vi "Read_raw_meas_setup.vi"(8 "Setup file string":string) -> (0 "No of Blocks":i32=1, 1 "Sampling freq (Hz)":dbl=100.0, 2 "No of samples":i32=500 min=0 step=1, 3 "Position":T2(array[cluster])=[{"Name"="LDA  (U)", "X"=3650.0, "Y"=0.0, "Z"=47.5}, {"Name"="Pitot 1 (Upitot)", "X"=3110.0, "Y"=0.0, "Z"=450.0}] {"Z" format="%.1f"; "Y" format="%.1f"; "X" format="%.1f"}, 5 "Correlate?":T1(ring))   [LabVIEW 2010]
uses:
  Globals/Meas_global.vi
  Globals/Trav_pos_global.vi
  Globals/LDA_meas_global_1.vi
  Globals/LDA_meas_global_2.vi
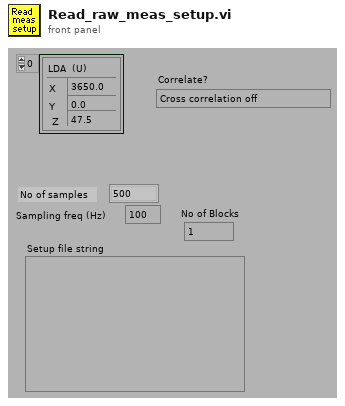
[diagram p1: front panel]
types:
  T1 = enum16{"Cross correlation off", "Show correlation panel", "Correlate without activating panel"}
  T2 = cluster{"Name":string, "X":dbl, "Y":dbl, "Z":dbl}[]
  T3 = typedef "Post_Process.ctl" = enum16{"Take New Data", "Post Process Raw Data File"}
  T4 = cluster{"Name":string, "X":dbl, "Y":dbl, "Z":dbl}
  T5 = enum16{"To Traverse Coordinates", "To User Coordinates"}
  T6 = enum16{"From String to Cluster", "From Cluster to String"}
  T7 = typedef "BSA_Type.ctl" = enum16{"57N11", "BSA F60"}
  T8 = typedef "BSA_info_Cluster.ctl" = cluster{"GPIB Address":string, "No of Check Bytes":i32, "Extra Info":string, "COLOUR":u32, "Wavelength (nm)":dbl}
  T9 = typedef "Tunnel_Coordinates.ctl" = enum16{"Work in Tunnel Coordinates", "Work in Model Coordinates"}
  T10 = typedef "Graph_Type.ctl" = enum16{"Show no graph", "Voltage trace", "Velocity trace", "Vel histogram", "Spectrum", "f.E(f) v Log f", "Auto-Corr"}
  T11 = cluster{"Plot 1":u16, "Plot 2":u16, "Save graph":u16, "Plot Type":T10}
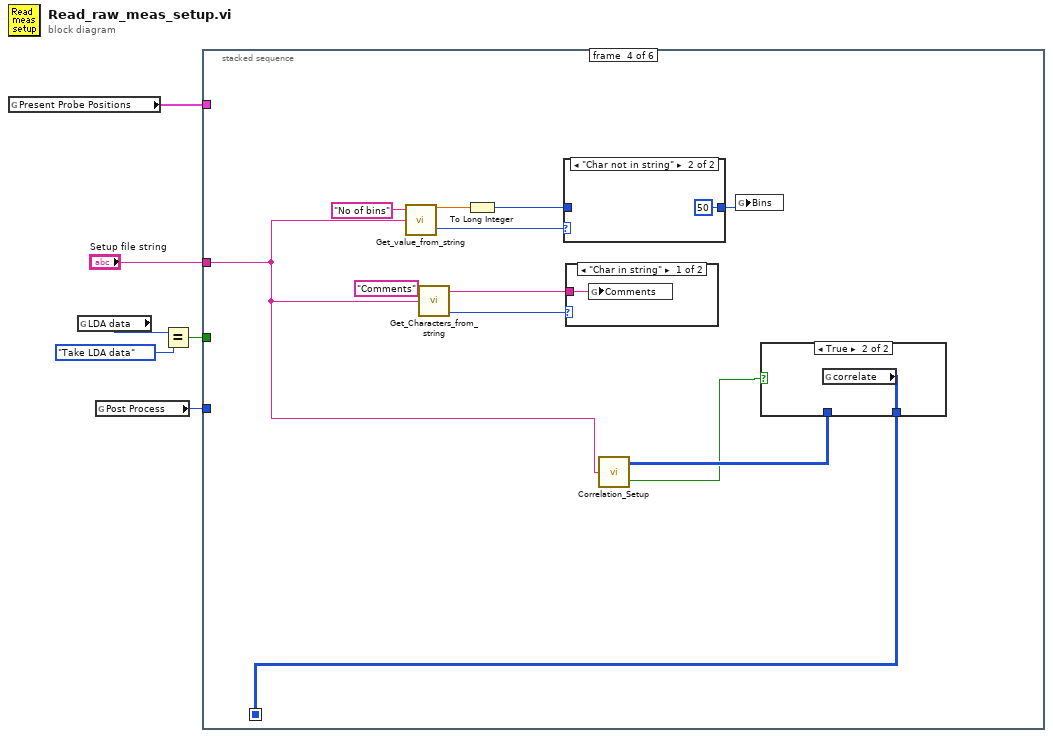
[diagram p0: block diagram]
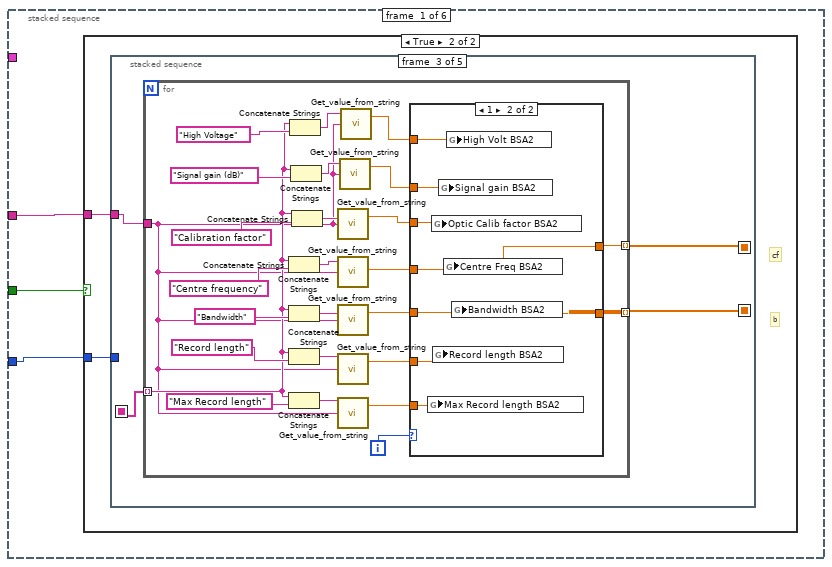
[diagram p2: hidden frame]
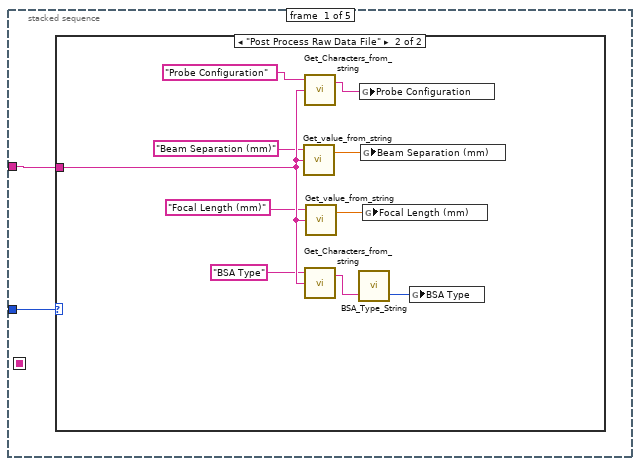
[diagram p4: hidden frame]
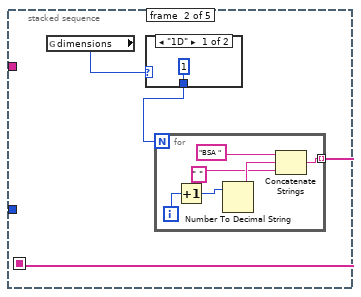
[diagram p6: hidden frame]
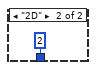
[diagram p7: hidden frame]
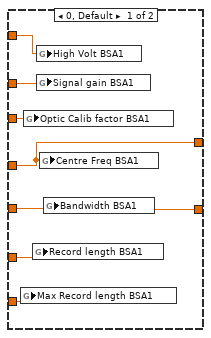
[diagram p8: hidden frame]
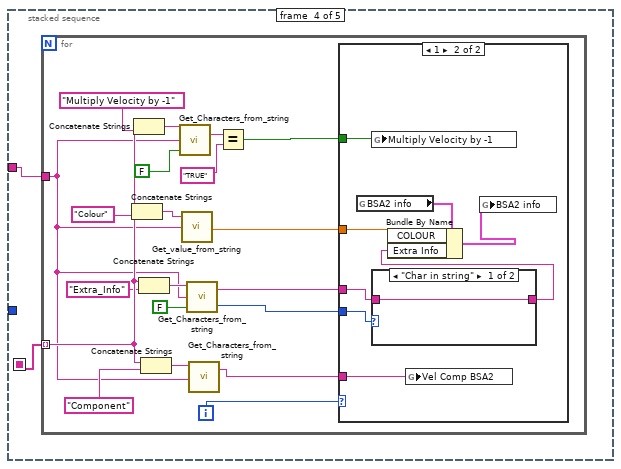
[diagram p9: hidden frame]
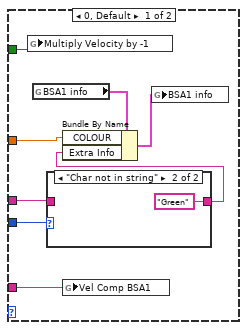
[diagram p10: hidden frame]
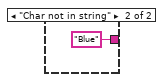
[diagram p12: hidden frame]
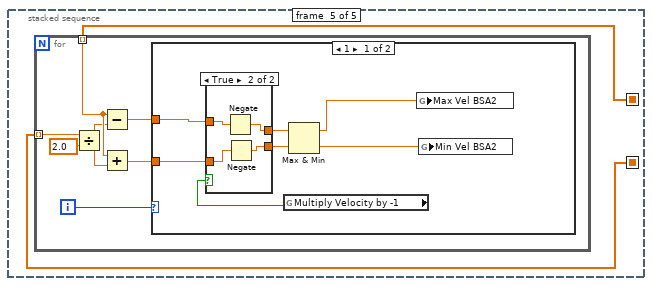
[diagram p13: hidden frame]
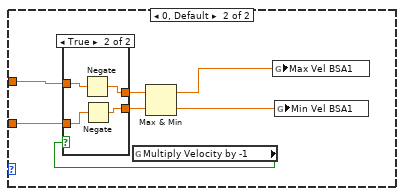
[diagram p15: hidden frame]
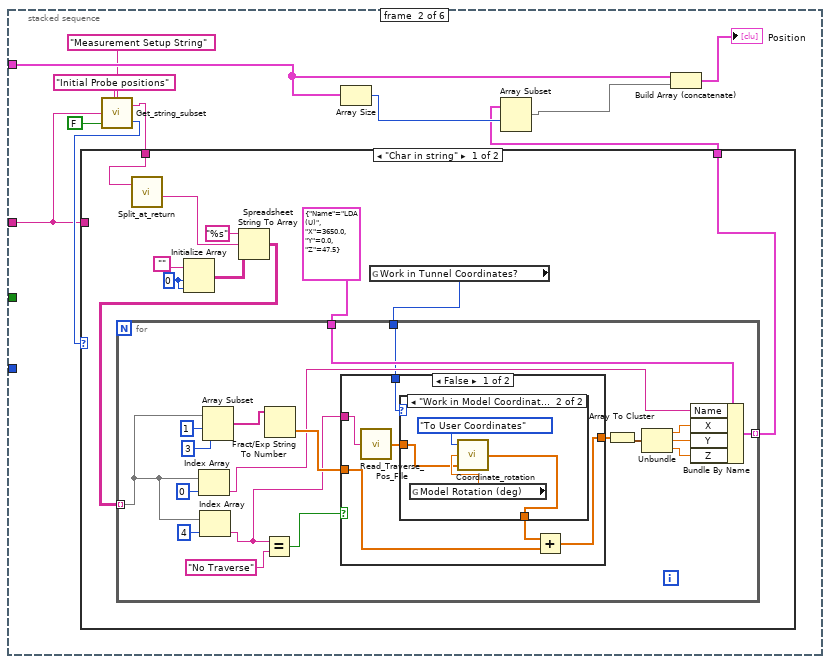
[diagram p17: hidden frame]
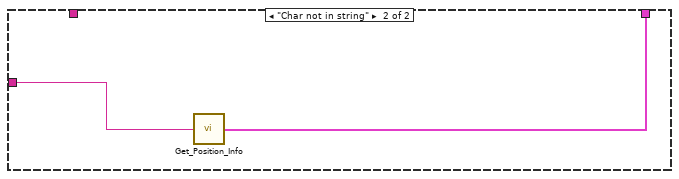
[diagram p20: hidden frame]
diagram:
  n1 = global read "Trav_pos_global.vi" "Present Probe Positions"() -> (w5:T2)
  n2 = global read "Meas_global.vi" "LDA data"() -> (w3:enum16{"No LDA data", "Take LDA data"})
  n3 = global read "Meas_global.vi" "Post Process"() -> (w6:T3)
  n4 = Equal?(x=w3, y=enum16{"No LDA data", "Take LDA data"}."Take LDA data" ("LDA data")) -> (x = y?=w2:bool)
  n5 = stacked-sequence {
    seq-local: [_ _ _ w226 _ _] -> [_ _ _ _ w245 _]
    tunnel: w6 -> [w7 _ _ _ _ _]
    tunnel: w5 -> [_ w165 _ _ _ _]
    tunnel: w2 -> [w9 _ _ _ _ _]
    tunnel: "Setup file string" -> [w8 w157 w215 w223 _ w248]
    frame #0 {
      n6 = case shown="True" w9 {
        tunnel: w8 -> [_ w11]
        tunnel: w7 -> [_ w10]
        frame False {
        }
        frame True {
          # "b"
          # "cf"
          n7 = stacked-sequence {
            seq-local: [_ w24 _ _ _] -> [_ _ w37 w79 _]
            seq-local: [_ _ w35 _ _] -> [_ _ _ _ w121]
            seq-local: [_ _ w36 _ _] -> [_ _ _ _ w122]
            tunnel: w11 -> [w12 _ w38 w80 _]
            tunnel: w10 -> [w13 _ _ _ _]
            frame #0 {
              n8 = case shown="\"Post Process Raw Data File\"" w13 {
                tunnel: w12 -> [_ w21]
                frame "Take New Data" {
                }
                frame "Post Process Raw Data File" {
                  n9 = call "Get_value_from_string.vi"("Input string"=w21, "Variable name"="Beam Separation (mm)" ("Label for characters")) -> ("Value"=w14:dbl)  [unwired: 1 in, 1 out]
                  n10 = call "Get_Characters_from_string.vi"("Input string"=w21, "Variable name"="Probe Configuration" ("Label for characters")) -> ("Value"=w22:string)  [unwired: 1 in, 1 out]
                  n11 = call "Get_Characters_from_string.vi"("Input string"=w21, "Variable name"="BSA Type" ("Label for characters")) -> ("Value"=w17:string)  [unwired: 1 in, 1 out]
                  n12 = call "Get_value_from_string.vi"("Input string"=w21, "Variable name"="Focal Length (mm)" ("Label for characters")) -> ("Value"=w15:dbl)  [unwired: 1 in, 1 out]
                  n13 = call "BSA_Type_String.vi"("BSA String in"=w17) -> ("BSA Type Out"=w16:T7)  [unwired: 1 in, 1 out]
                  n14 = global write "LDA_meas_global_1.vi" "Probe Configuration"(w22) -> ()
                  n15 = global write "LDA_meas_global_1.vi" "Beam Separation (mm)"(w14) -> ()
                  n16 = global write "LDA_meas_global_1.vi" "Focal Length (mm)"(w15) -> ()
                  n17 = global write "LDA_meas_global_1.vi" "BSA Type"(w16) -> ()
                }
              }
            }
            frame #1 {
              n18 = global read "Meas_global.vi" "dimensions"() -> (w26:enum16{"1D", "2D"})
              n19 = case shown="\"1D\"" w26 {
                tunnel: [1 2] -> w25
                frame "1D" {
                }
                frame "2D" {
                }
              }
              n20 = for {
                N: w25 -> [_]
                tunnel: [w28] -> w24 mode=indexing
                i -> [w30]
                n21 = Increment(x=w30) -> (x+1=w29:i32)
                n22 = Number To Decimal String(number=w29) -> (decimal integer string=w32:string)  [unwired: 1 out]
                n23 = Concatenate Strings("BSA ", w32, " ") -> (w28:string)
              }
            }
            frame #2 {
              n24 = for {
                tunnel: w38 -> [w39]
                tunnel: w37 -> [w40] mode=indexing
                tunnel: [w52] -> w36 mode=indexing
                tunnel: [w51] -> w35 mode=indexing
                i -> [w56]
                n25 = Concatenate Strings(w40, "Centre frequency") -> (w59:string)
                n26 = Concatenate Strings(w40, "Bandwidth") -> (w58:string)
                n27 = Concatenate Strings(w40, "Record length") -> (w57:string)
                n28 = Concatenate Strings(w40, "Max Record length") -> (w42:string)
                n29 = Concatenate Strings(w40, "High Voltage") -> (w46:string)
                n30 = Concatenate Strings(w40, "Signal gain (dB)") -> (w47:string)
                n31 = Concatenate Strings(w40, "Calibration factor") -> (w60:string)
                n32 = call "Get_value_from_string.vi"("Input string"=w39, "Variable name"=w60) -> ("Value"=w50:dbl)  [unwired: 1 in, 1 out]
                n33 = call "Get_value_from_string.vi"("Input string"=w39, "Variable name"=w59) -> ("Value"=w55:dbl)  [unwired: 1 in, 1 out]
                n34 = call "Get_value_from_string.vi"("Input string"=w39, "Variable name"=w58) -> ("Value"=w54:dbl)  [unwired: 1 in, 1 out]
                n35 = call "Get_value_from_string.vi"("Input string"=w39, "Variable name"=w57) -> ("Value"=w53:dbl)  [unwired: 1 in, 1 out]
                n36 = call "Get_value_from_string.vi"("Input string"=w39, "Variable name"=w42) -> ("Value"=w43:dbl)  [unwired: 1 in, 1 out]
                n37 = call "Get_value_from_string.vi"("Input string"=w39, "Variable name"=w47) -> ("Value"=w45:dbl)  [unwired: 1 in, 1 out]
                n38 = call "Get_value_from_string.vi"("Input string"=w39, "Variable name"=w46) -> ("Value"=w44:dbl)  [unwired: 1 in, 1 out]
                n39 = case shown="1" w56 {
                  tunnel: w55 -> [w68 w76]
                  tunnel: w54 -> [w69 w75]
                  tunnel: w53 -> [w70 w78]
                  tunnel: w50 -> [w71 w77]
                  tunnel: [w69 w75] -> w52
                  tunnel: [w68 w76] -> w51
                  tunnel: w45 -> [w67 w73]
                  tunnel: w44 -> [w66 w74]
                  tunnel: w43 -> [w65 w72]
                  frame 0, Default {
                    n40 = global write "LDA_meas_global_1.vi" "Max Record length BSA1"(w65) -> ()
                    n41 = global write "LDA_meas_global_1.vi" "Optic Calib factor BSA1"(w71) -> ()
                    n42 = global write "LDA_meas_global_1.vi" "Record length BSA1"(w70) -> ()
                    n43 = global write "LDA_meas_global_1.vi" "High Volt BSA1"(w66) -> ()
                    n44 = global write "LDA_meas_global_1.vi" "Signal gain BSA1"(w67) -> ()
                    n45 = global write "LDA_meas_global_1.vi" "Centre Freq BSA1"(w68) -> ()
                    n46 = global write "LDA_meas_global_1.vi" "Bandwidth BSA1"(w69) -> ()
                  }
                  frame 1 {
                    n47 = global write "LDA_meas_global_2.vi" "Max Record length BSA2"(w72) -> ()
                    n48 = global write "LDA_meas_global_2.vi" "Optic Calib factor BSA2"(w77) -> ()
                    n49 = global write "LDA_meas_global_2.vi" "Record length BSA2"(w78) -> ()
                    n50 = global write "LDA_meas_global_2.vi" "Signal gain BSA2"(w73) -> ()
                    n51 = global write "LDA_meas_global_2.vi" "Centre Freq BSA2"(w76) -> ()
                    n52 = global write "LDA_meas_global_2.vi" "High Volt BSA2"(w74) -> ()
                    n53 = global write "LDA_meas_global_2.vi" "Bandwidth BSA2"(w75) -> ()
                  }
                }
              }
            }
            frame #3 {
              n54 = for {
                tunnel: w80 -> [w81]
                tunnel: w79 -> [w86] mode=indexing
                i -> [w98]
                n55 = Concatenate Strings(w86, "Colour") -> (w99:string)
                n56 = Concatenate Strings(w86, "Multiply Velocity by -1") -> (w92:string)
                n57 = Concatenate Strings(w86, "Extra_Info" ("string")) -> (w87:string)
                n58 = Concatenate Strings(w86, "Component") -> (w100:string)
                n59 = call "Get_Characters_from_string.vi"("Show Dialog?"=FALSE, "Input string"=w81, "Variable name"=w92) -> ("Value"=w90:string)  [unwired: 1 out]
                n60 = call "Get_value_from_string.vi"("Input string"=w81, "Variable name"=w99) -> ("Value"=w95:dbl)  [unwired: 1 in, 1 out]
                n61 = call "Get_Characters_from_string.vi"("Show Dialog?"=FALSE, "Input string"=w81, "Variable name"=w87) -> ("Status"=w83:enum16{"Char in string", "Char not in string"}, "Value"=w82:string)
                n62 = call "Get_Characters_from_string.vi"("Input string"=w81, "Variable name"=w100) -> ("Value"=w94:string)  [unwired: 1 in, 1 out]
                n63 = Equal?(x=w90, y="TRUE") -> (x = y?=w88:bool)
                n64 = case shown="1" w98 {
                  tunnel: w95 -> [w107 w117]
                  tunnel: w94 -> [w106 w116]
                  tunnel: w88 -> [w105 w115]
                  tunnel: w83 -> [w104 w112]
                  tunnel: w82 -> [w103 w113]
                  frame 0, Default {
                    n65 = global write "LDA_meas_global_1.vi" "Multiply Velocity by -1"(w105) -> ()
                    n66 = global read "LDA_meas_global_1.vi" "BSA1 info"() -> (w108:T8)
                    n67 = case shown="\"Char not in string\"" w104 {
                      tunnel: w103 -> [w109 _]
                      tunnel: [w109 "Green" ("Value")] -> w101
                      frame "Char in string" {
                      }
                      frame "Char not in string" {
                      }
                    }
                    n68 = Bundle By Name(cluster=w108, "COLOUR"=w107, "Extra Info"=w101) -> (w102:T8)
                    n69 = global write "LDA_meas_global_1.vi" "Vel Comp BSA1"(w106) -> ()
                    n70 = global write "LDA_meas_global_1.vi" "BSA1 info"(w102) -> ()
                  }
                  frame 1 {
                    n71 = global read "LDA_meas_global_2.vi" "BSA2 info"() -> (w118:T8)
                    n72 = global write "LDA_meas_global_2.vi" "Multiply Velocity by -1"(w115) -> ()
                    n73 = case shown="\"Char in string\"" w112 {
                      tunnel: w113 -> [w119 _]
                      tunnel: [w119 "Blue" ("Value")] -> w111
                      frame "Char in string" {
                      }
                      frame "Char not in string" {
                      }
                    }
                    n74 = Bundle By Name(cluster=w118, "COLOUR"=w117, "Extra Info"=w111) -> (w114:T8)
                    n75 = global write "LDA_meas_global_2.vi" "Vel Comp BSA2"(w116) -> ()
                    n76 = global write "LDA_meas_global_2.vi" "BSA2 info"(w114) -> ()
                  }
                }
              }
            }
            frame #4 {
              n77 = for {
                tunnel: w122 -> [w128] mode=indexing
                tunnel: w121 -> [w127] mode=indexing
                i -> [w123]
                n78 = Divide(x=w128, y=2.0) -> (x/y=w126:dbl)
                n79 = Subtract(x=w127, y=w126) -> (x-y=w124:dbl)
                n80 = Add(x=w127, y=w126) -> (x+y=w125:dbl)
                n81 = case shown="1" w123 {
                  tunnel: w125 -> [w136 w149]
                  tunnel: w124 -> [w135 w148]
                  frame 1 {
                    n82 = global read "LDA_meas_global_2.vi" "Multiply Velocity by -1"() -> (w132:bool)
                    n83 = case shown="True" w132 {
                      tunnel: w136 -> [w137 w142]
                      tunnel: w135 -> [w138 w141]
                      tunnel: [w138 w140] -> w134
                      tunnel: [w137 w139] -> w133
                      frame False {
                      }
                      frame True {
                        n84 = Negate(x=w141) -> (-x=w140:dbl)
                        n85 = Negate(x=w142) -> (-x=w139:dbl)
                      }
                    }
                    n86 = Max & Min(x=w134, y=w133) -> (max(x,y)=w130:dbl, min(x,y)=w131:dbl)
                    n87 = global write "LDA_meas_global_2.vi" "Max Vel BSA2"(w130) -> ()
                    n88 = global write "LDA_meas_global_2.vi" "Min Vel BSA2"(w131) -> ()
                  }
                  frame 0, Default {
                    n89 = global read "LDA_meas_global_1.vi" "Multiply Velocity by -1"() -> (w145:bool)
                    n90 = case shown="True" w145 {
                      tunnel: w149 -> [w150 w155]
                      tunnel: w148 -> [w151 w154]
                      tunnel: [w151 w153] -> w147
                      tunnel: [w150 w152] -> w146
                      frame False {
                      }
                      frame True {
                        n91 = Negate(x=w154) -> (-x=w153:dbl)
                        n92 = Negate(x=w155) -> (-x=w152:dbl)
                      }
                    }
                    n93 = Max & Min(x=w147, y=w146) -> (max(x,y)=w143:dbl, min(x,y)=w144:dbl)
                    n94 = global write "LDA_meas_global_1.vi" "Max Vel BSA1"(w143) -> ()
                    n95 = global write "LDA_meas_global_1.vi" "Min Vel BSA1"(w144) -> ()
                  }
                }
              }
            }
          }
        }
      }
    }
    frame #1 {
      n96 = call "Get_string_subset.vi"("String Name"="Measurement Setup String", "Show Dialog?"=FALSE, "String to split"=w157, "File Label"="Initial Probe positions") -> ("Status"=w162:enum16{"Char in string", "Char not in string"}, "Output string"=w161:string)
      n97 = case shown="\"Char in string\"" w162 {
        tunnel: w161 -> [w172 _]
        tunnel: w157 -> [_ w209]
        tunnel: [w168 w208] -> w159
        frame "Char in string" {
          w175 = 0 ("Dimension Size")
          n98 = call "Split_at_return.vi"("String"=w172) -> ("after substring"=w171:string)  [unwired: 1 in, 3 out]
          n99 = Initialize Array("", w175, w175) -> (w176:string[][])
          n100 = Spreadsheet String To Array(format string="%s", spreadsheet string=w171, array type (2D Dbl)=w176) -> (array=w170:string[][])  [unwired: 1 out]
          n101 = global read "Trav_pos_global.vi" "Work in Tunnel Coordinates?"() -> (w167:T9)
          n102 = for {
            tunnel: w170 -> [w181] mode=indexing
            tunnel: T4 {"Name"="LDA  (U)", "X"=3650.0, "Y"=0.0, "Z"=47.5} ("Position") -> [w195]
            tunnel: [w179] -> w168 mode=indexing
            tunnel: w167 -> [w177]
            n103 = Index Array(array=w181, index=0) -> (element=w180:string)
            n104 = Index Array(array=w181, index=4) -> (element=w178:string)
            n105 = Array Subset(array=w181, index=1, length=3) -> (w191:string[])
            n106 = Equal?(x=w178, y="No Traverse" ("x")) -> (x = y?=w190:bool)
            n107 = Fract/Exp String To Number(string=w191) -> (number=w188:dbl[])  [unwired: 4 out]
            n108 = case shown="False" w190 {
              tunnel: [w200 w207] -> w189
              tunnel: w188 -> [w201 w207]
              tunnel: w178 -> [w199 _]
              tunnel: w177 -> [w198 _]
              frame False {
                n109 = call "Read_Traverse_Pos_File.vi"("Traverse Name"=w199) -> ("Tunnel Coordinates"=w196:dbl[])
                n110 = case shown="\"Work in Model Coordinates\"" w198 {
                  tunnel: [w202 w203] -> w197
                  tunnel: w196 -> [w202 w204]
                  frame "Work in Tunnel Coordinates" {
                  }
                  frame "Work in Model Coordinates" {
                    n111 = global read "Trav_pos_global.vi" "Model Rotation (deg)"() -> (w205:dbl)
                    n112 = call "Coordinate_rotation.vi"("Input Position"=w204, "Coordinate rotation (deg)"=w205, "Mode"=T5."To User Coordinates") -> ("Output Position"=w203:dbl[])
                  }
                }
                n113 = Add(x=w197, y=w201) -> (x+y=w200:dbl[])
              }
              frame True {
              }
            }
            n114 = Array To Cluster(array=w189) -> (cluster=w187:cluster{"[0]":dbl, "[1]":dbl, "[2]":dbl})
            n115 = Unbundle(w187) -> ("[0]"=w186:dbl, "[1]"=w185:dbl, "[2]"=w184:dbl)
            n116 = Bundle By Name(cluster=w195, "Name"=w180, "X"=w186, "Y"=w185, "Z"=w184) -> (w179:T4)
          }
        }
        frame "Char not in string" {
          n117 = call "Get_Position_Info.vi"("Input string"=w209) -> ("Position"=w208:T2)
        }
      }
      n118 = Array Size(array=w165) -> (size(s)=w160:i32)
      n119 = Array Subset(array=w159, index=w160) -> (w158:T2)  [unwired: 1 in]
      n120 = Build Array (concatenate)(w165, w158) -> (→"Position":T2)
    }
    frame #2 {
      n121 = call "Get_value_from_string.vi"("Input string"=w215, "Variable name"="No of samples") -> ("Value"=→"No of samples":dbl)  [unwired: 1 in, 1 out]
      n122 = call "Get_value_from_string.vi"("Input string"=w215, "Variable name"="Requested sampling rate") -> ("Status"=w213:enum16{"Char in string", "Char not in string"}, "Value"=w211:dbl)  [unwired: 1 in]
      n123 = call "Get_value_from_string.vi"("Input string"=w215, "Variable name"="Actual sampling rate") -> ("Value"=w210:dbl)  [unwired: 1 in, 1 out]
      n124 = call "Get_value_from_string.vi"("Input string"=w215, "Variable name"="No of blocks") -> ("Value"=→"No of Blocks":dbl)  [unwired: 1 in, 1 out]
      n125 = global write "Meas_global.vi" "Actual Sampling rate (Hz)"(w210) -> ()
      n126 = case shown="\"Char not in string\"" w213 {
        tunnel: [w221 w222] -> w212
        tunnel: w211 -> [w221 _]
        tunnel: w210 -> [_ w222]
        frame "Char in string" {
        }
        frame "Char not in string" {
        }
      }
      "Sampling freq (Hz)" <- w212
    }
    frame #3 {
      n127 = call "Get_value_from_string.vi"("Input string"=w223, "Variable name"="No of bins") -> ("Status"=w233:enum16{"Char in string", "Char not in string"}, "Value"=w232:dbl)  [unwired: 1 in]
      n128 = call "Get_Characters_from_string.vi"("Input string"=w223, "Variable name"="Comments") -> ("Status"=w230:enum16{"Char in string", "Char not in string"}, "Value"=w229:string)  [unwired: 1 in]
      n129 = To Long Integer(number=w232) -> (32bit integer=w231:i32)
      n130 = case shown="\"Char not in string\"" w233 {
        tunnel: w231 -> [w238 _]
        tunnel: [w238 50] -> w227
        frame "Char in string" {
        }
        frame "Char not in string" {
        }
      }
      n131 = case shown="\"Char in string\"" w230 {
        tunnel: w229 -> [w237 _]
        frame "Char in string" {
          n132 = global write "Meas_global.vi" "Comments"(w237) -> ()
        }
        frame "Char not in string" {
        }
      }
      n133 = call "Correlation_Setup.vi"("Input string"=w223) -> ("Correlate"=w225:i32[][], "Error?"=w224:bool)
      n134 = global write "Meas_global.vi" "Bins"(w227) -> ()
      n135 = case shown="True" w224 {
        tunnel: w225 -> [w235 _]
        tunnel: [w235 w236] -> w226
        frame False {
          n136 = global write "Meas_global.vi" "correlate"(w235) -> ()
        }
        frame True {
          n137 = global read "Meas_global.vi" "correlate"() -> (w236:i32[][])
        }
      }
    }
    frame #4 {
      n138 = Array Size(array=w245) -> (size(s)=w247:i32[])
      n139 = Index Array(array=w247, index=0) -> (element=w244:i32)
      n140 = Equal To 0?(x=w244) -> (x = 0?=w240:bool)
      n141 = Select(t=T1."Cross correlation off" ("Correlate?"), s=w240, f=T1."Correlate without activating panel" ("Correlate?")) -> (s? t:f=→"Correlate?":T1)
    }
    frame #5 {
      n142 = call "Save_Load_Graph_Setup.vi"("Setup String in"=w248, "Graph Number"=1, "Mode"=T6."From String to Cluster") -> ("Variables found?"=w254:bool, "Graph Out"=w253:T11)  [unwired: 1 in, 1 out]
      n143 = call "Save_Load_Graph_Setup.vi"("Setup String in"=w248, "Graph Number"=2, "Mode"=T6."From String to Cluster") -> ("Variables found?"=w250:bool, "Graph Out"=w249:T11)  [unwired: 1 in, 1 out]
      n144 = case shown="True" w254 {
        tunnel: w253 -> [_ w258]
        frame False {
        }
        frame True {
          n145 = global write "Meas_global.vi" "First Graph"(w258) -> ()
        }
      }
      n146 = case shown="True" w250 {
        tunnel: w249 -> [_ w257]
        frame False {
        }
        frame True {
          n147 = global write "Meas_global.vi" "Second Graph"(w257) -> ()
        }
      }
    }
  }
